vi "BallShear_main.vi"() -> ()   [LabVIEW 2013]
panel:
  out "Livefeed":path
  out "Ball_Detection":path
  out "Coord_Conversion":path
  out "VCoord":path
  out "RCoord":path
  out "Force Reading":path
  out "Analyzed Image":path
  out "Package Image":path
  out "Default Image":path
  in  "Array":dbl[][](array[numeric])
  out "Selected \nCoordinates":dbl[][](array[numeric])
  out "Selected Indices":dbl[](array[numeric])
  out "Coordinates":dbl[][](array[numeric])
  out "Ball IDs":string[](array[string])
  out "Current Step":i32
  in  "Options":enum32{"Shear", "Results", "Settings"}(tab)
  out "Status":string
  out "# Balls Selected":dbl
  in  "Shear Speed":dbl=1.0 min=1.0 max=2.0 step=0.01 format="%#_6f"
  out "Total Steps":dbl
  in  "Check":bool
  out "Ready":bool
  in  "Remove Package":bool
  in  "Proceed":bool
  in  "Preceed":bool
  out "Step":dbl
  out "Package":picture
  in  "Ball Selection":i32[](listbox)
  in  "Max Shear Speed":dbl
  in  "Min Shear Speed":dbl
  in  "Image Path":path
  in  "Image Name":string
  out "Displayed Image":path=path "C:/Users/nsliwa/Documents/GitHub/Ball_Shear/Images/default.jpg"
  in  "Image Path":string
  out "Ready":bool
  in  "Power":bool=TRUE
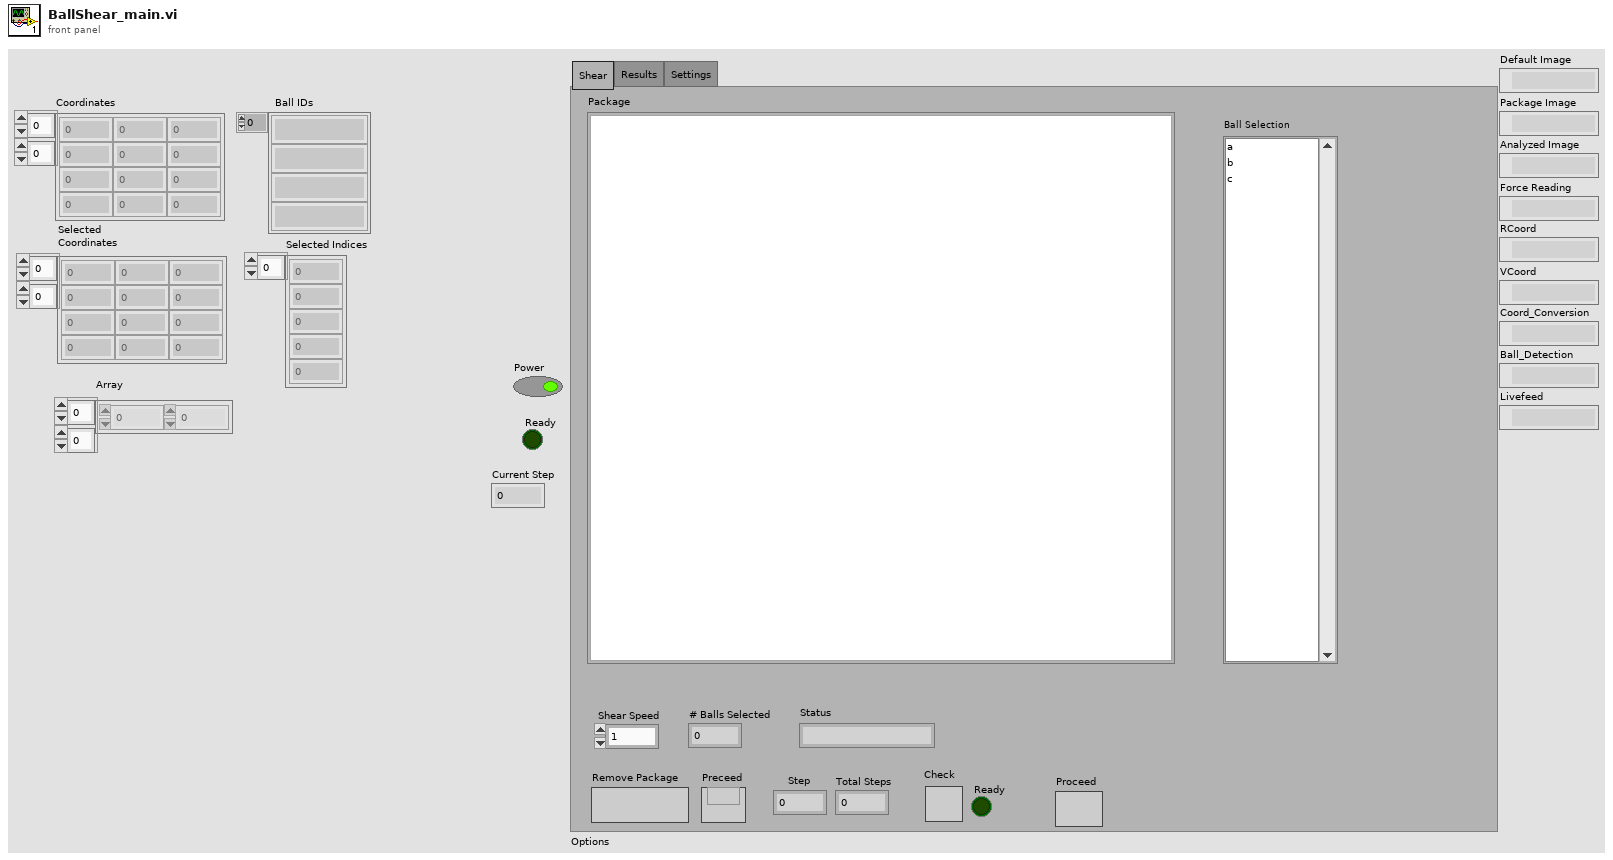
[diagram p1: front panel]
types:
  T1 = typedef "imagedata.ctl" = cluster{"image type":i32, "image depth":i32, "image":u8[], "mask":u8[], "colors":u32[], "Rectangle":cluster{"left":i16, "top":i16, "right":i16, "bottom":i16}}
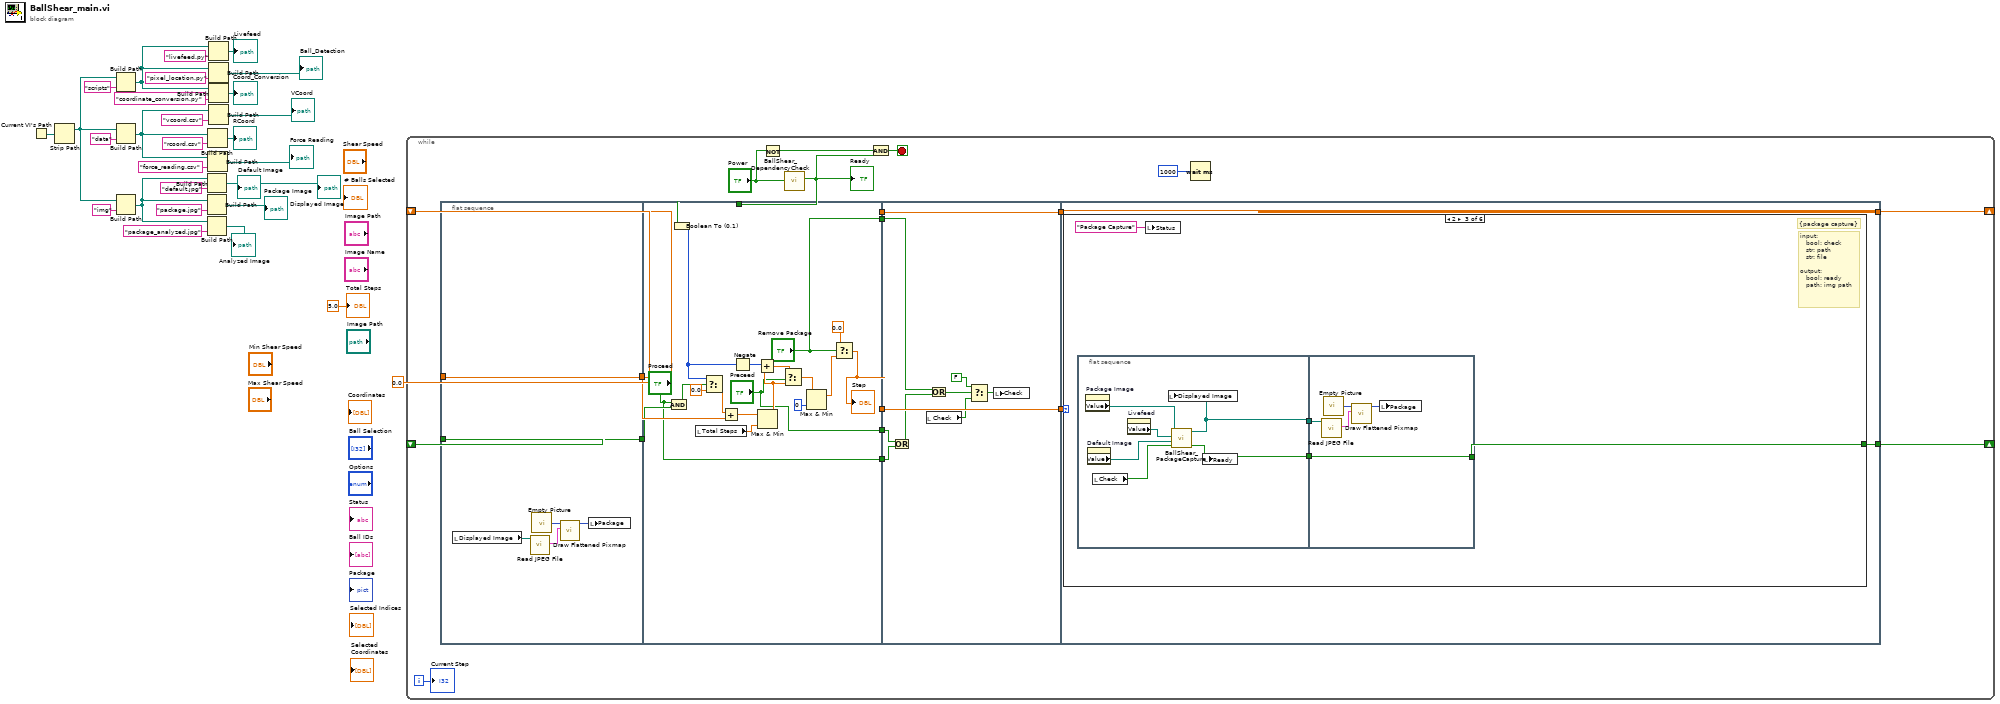
[diagram p0: block diagram]
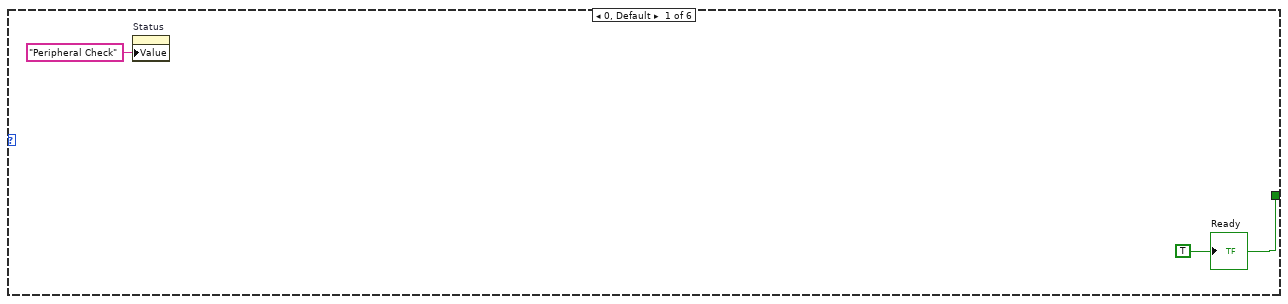
[diagram p2: hidden frame]
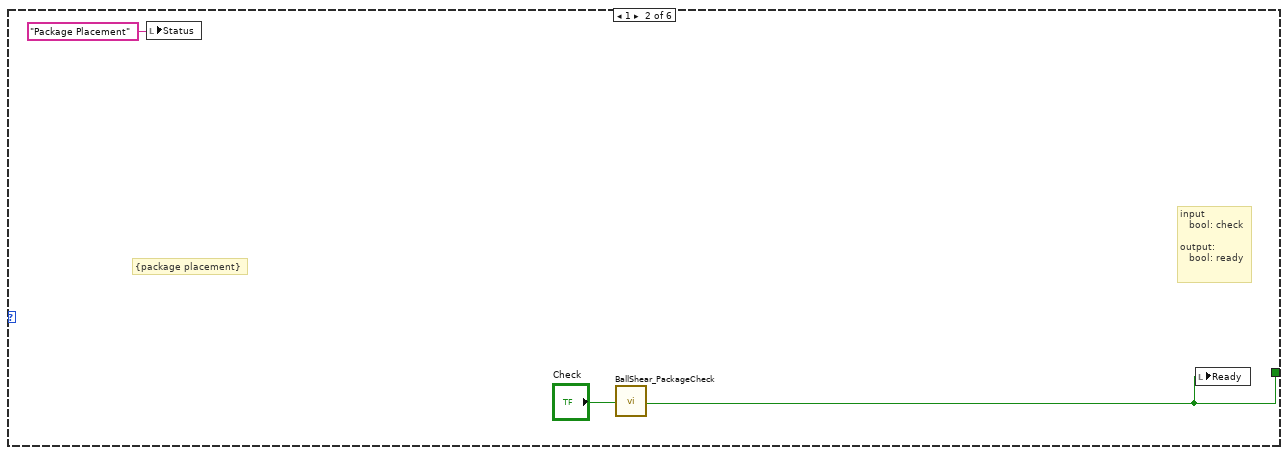
[diagram p3: hidden frame]
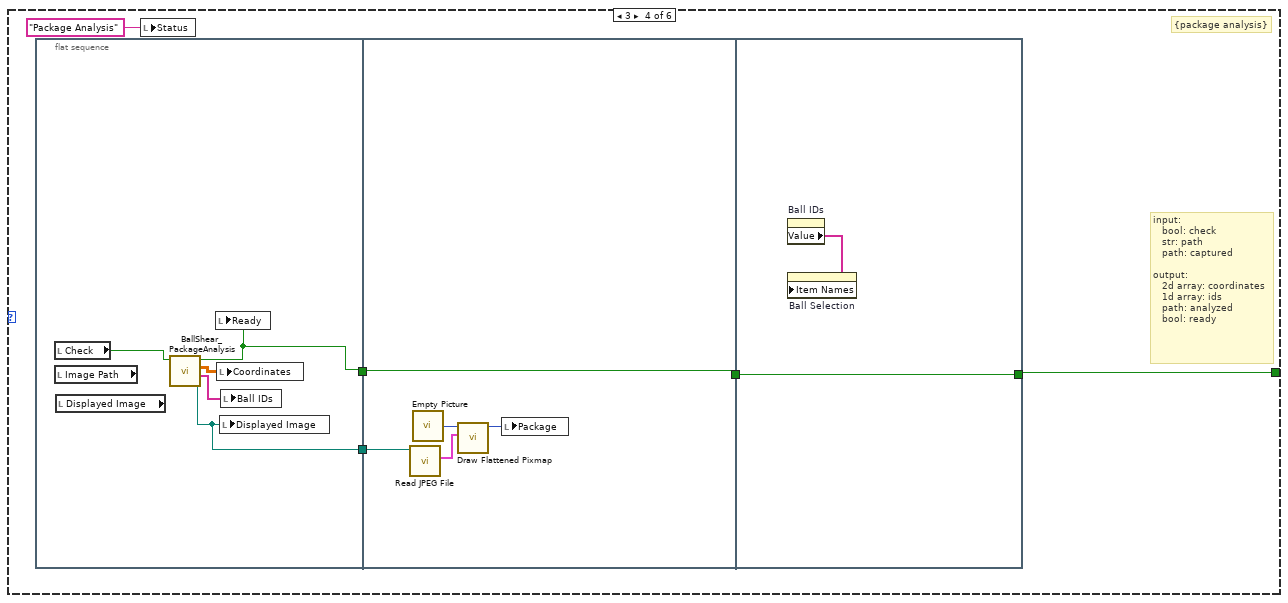
[diagram p4: hidden frame]
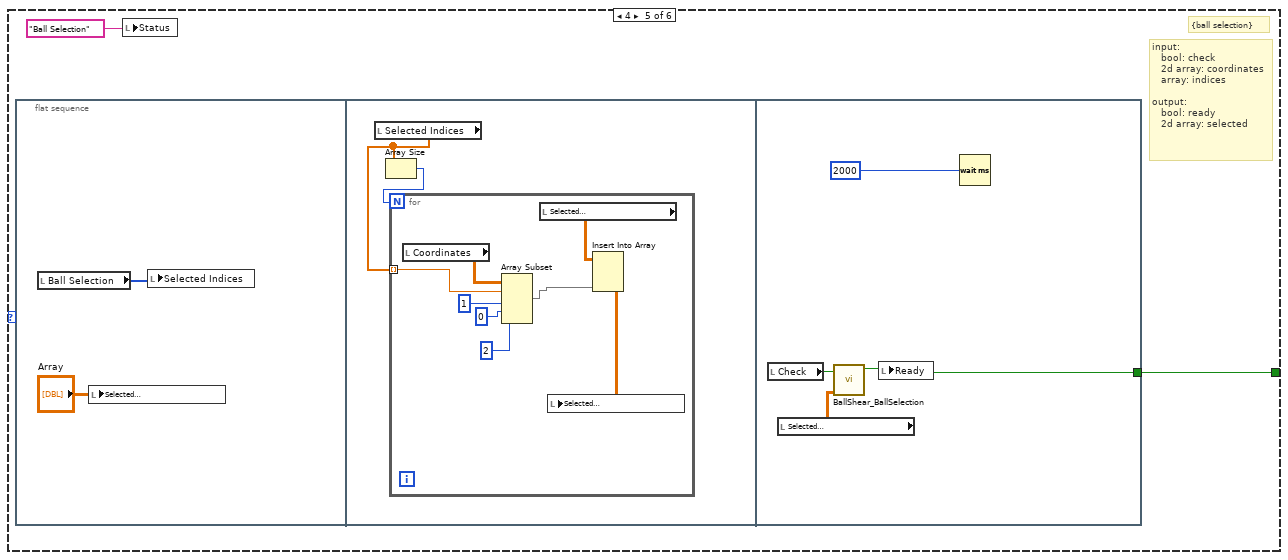
[diagram p5: hidden frame]
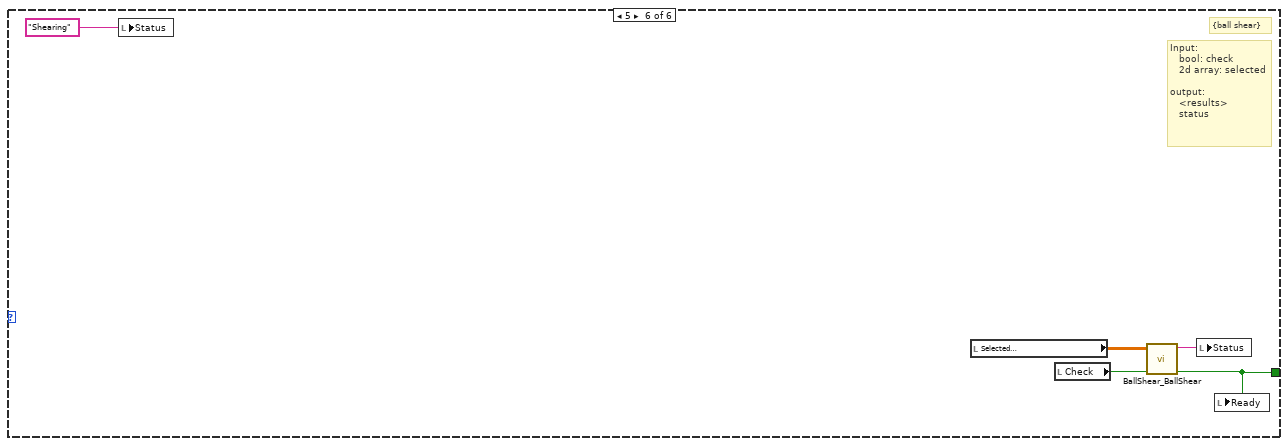
[diagram p6: hidden frame]
diagram:
  n1 = Current VI's Path() -> (path=w26:path)
  n2 = Strip Path(path=w26) -> (stripped path=w24:path)  [unwired: 1 out]
  n3 = Build Path(base path=w24, name or relative path="scripts") -> (appended path=w20:path)
  n4 = Build Path(base path=w24, name or relative path="data") -> (appended path=w15:path)
  n5 = Build Path(base path=w24, name or relative path="img") -> (appended path=w21:path)
  n6 = Build Path(base path=w21, name or relative path="default.jpg") -> (appended path=→"Displayed Image" →"Default Image":path)
  n7 = Build Path(base path=w21, name or relative path="package.jpg") -> (appended path=→"Package Image":path)
  n8 = Build Path(base path=w21, name or relative path="package_analyzed.jpg") -> (appended path=→"Analyzed Image":path)
  n9 = Build Path(base path=w15, name or relative path="rcoord.csv") -> (appended path=→"RCoord":path)
  n10 = Build Path(base path=w15, name or relative path="force_reading.csv") -> (appended path=→"Force Reading":path)
  n11 = Build Path(base path=w20, name or relative path="livefeed.py") -> (appended path=→"Livefeed":path)
  n12 = Build Path(base path=w20, name or relative path="pixel_location.py") -> (appended path=→"Ball_Detection":path)
  n13 = Build Path(base path=w20, name or relative path="coordinate_conversion.py") -> (appended path=→"Coord_Conversion":path)
  n14 = Build Path(base path=w15, name or relative path="vcoord.csv") -> (appended path=→"VCoord":path)
  n15 = while {
    shift-right: [w40] -> _
    shift-left: 0.0 ("Step") -> [w42]
    shift-right: [w38] -> _
    shift-left: _ -> [w36]
    i -> [w43]
    stop <- w45 stop-if-true
    n16 = flat-sequence {
      tunnel: w42 -> [w53]
      tunnel: [w53] -> w39
      tunnel: [w52] -> w37
      tunnel: w36 -> [w52]
      tunnel: w41 -> [w68]
      tunnel: [w59] -> w35
      tunnel: w39 -> [w69]
      tunnel: [w59] -> w33
      tunnel: w37 -> [w58]
      tunnel: ["Remove Package"] -> w31
      tunnel: ["Proceed"] -> w30
      tunnel: ["Preceed"] -> w29
      tunnel: w35 -> [w83]
      tunnel: [w83] -> w34
      tunnel: w33 -> [w82]
      tunnel: [w82] -> w32
      tunnel: w31 -> [w79]
      tunnel: w30 -> [w80]
      tunnel: w29 -> [w81]
      tunnel: [w86] -> w40
      tunnel: w34 -> [w86]
      tunnel: w32 -> [w85]
      tunnel: [w84] -> w38
      frame #0 {
        n17 = local read "Displayed Image"() -> (w48:path)
        n18 = call <vilib>:"Read JPEG File.vi"("path to JPEG file"=w48) -> ("image data"=w49:T1)  [unwired: 8 in, 2 out]
        n19 = call "Empty Picture"() -> ("empty picture"=w50:picture)
        n20 = call <vilib>:"Draw Flattened Pixmap.vi"("image data"=w49, "picture"=w50) -> ("new picture"=w51:picture)  [unwired: 7 in]
        n21 = local write "Package"(w51) -> ()
      }
      frame #1 {
        n22 = And(x="Proceed", y=w58) -> (x .and. y?=w57:bool)
        n23 = Boolean To (0,1)(Boolean=w68) -> (0, 1=w67:i16)
        n24 = local read "Total Steps"() -> (w61:dbl)
        n25 = Select(t=w67, s=w57, f=0.0) -> (s? t:f=w71:dbl)
        n26 = Add(x=w71, y=w69) -> (x+y=w66:dbl)
        n27 = Negate(x=w67) -> (-x=w72:i16)
        n28 = Max & Min(x=w66, y=w61) -> (min(x,y)=w65:dbl)  [unwired: 1 out]
        n29 = Add(x=w72, y=w65) -> (x+y=w73:dbl)
        n30 = Select(t=w73, s="Preceed", f=w65) -> (s? t:f=w64:dbl)
        n31 = Max & Min(x=w64, y=i16 0) -> (max(x,y)=w63:dbl)  [unwired: 1 out]
        n32 = Select(t=0.0, s="Remove Package", f=w63) -> (s? t:f=w59:dbl)
        "Step" <- w59
      }
      frame #2 {
        n33 = Or(x=w81, y=w80) -> (x .or. y?=w78:bool)
        n34 = local read "Check"() -> (w75:bool)
        n35 = Or(x=w79, y=w78) -> (x .or. y?=w77:bool)
        n36 = Select(t=FALSE, s=w77, f=w75) -> (s? t:f=w74:bool)
        n37 = local write "Check"(w74) -> ()
      }
      frame #3 {
        n38 = case shown="2" w85 {
          tunnel: [w88 w90 w94 w110 w124 w144] -> w84
          frame 0, Default {
            w88 = TRUE
            n39 = property on="Status" class="Str"("Value"="Peripheral Check" ("Status")) -> ()  [unwired: 2 in, 2 out]
            "Ready" <- w88
          }
          frame 1 {
            # "input\n   bool: check\n\noutput:\n   bool: ready"
            # "{package placement}"
            n40 = local write "Status"("Package Placement" ("Status")) -> ()
            n41 = call "BallShear_PackageCheck.vi"("Check"="Check") -> ("Ready"=w90:bool)  [unwired: 10 in]
            n42 = local write "Ready"(w90) -> ()
          }
          frame 2 {
            # "input: \n   bool: check\n   str: path\n   str: file\n\noutput:\n   bool: ready\n   path: img path"
            # "{package capture}"
            n43 = flat-sequence {
              tunnel: [w101] -> w93
              tunnel: [w100] -> w92
              tunnel: w93 -> [w106]
              tunnel: w92 -> [w103]
              tunnel: [w106] -> w94
              frame #0 {
                n44 = property on="Package Image" class="Path"() -> ("Value"=w98:path)  [unwired: 2 in, 2 out]
                n45 = property on="Default Image" class="Path"() -> ("Value"=w96:path)  [unwired: 2 in, 2 out]
                n46 = local read "Check"() -> (w99:bool)
                n47 = property on="Livefeed" class="Path"() -> ("Value"=w97:path)  [unwired: 2 in, 2 out]
                n48 = call "BallShear_PackageCapture.vi"("Capture"=w99, "Default Image Path"=w96, "Python Script Path"=w97, "Target Image Path"=w98) -> ("Success"=w101:bool, "Actual Image Path"=w100:path)  [unwired: 6 in]
                n49 = local write "Displayed Image"(w100) -> ()
                n50 = local write "Ready"(w101) -> ()
              }
              frame #1 {
                n51 = call <vilib>:"Read JPEG File.vi"("path to JPEG file"=w103) -> ("image data"=w105:T1)  [unwired: 8 in, 2 out]
                n52 = call "Empty Picture"() -> ("empty picture"=w104:picture)
                n53 = call <vilib>:"Draw Flattened Pixmap.vi"("image data"=w105, "picture"=w104) -> ("new picture"=w102:picture)  [unwired: 7 in]
                n54 = local write "Package"(w102) -> ()
              }
            }
            n55 = local write "Status"("Package Capture" ("Status")) -> ()
          }
          frame 3 {
            # "input:\n   bool: check\n   str: path\n   path: captured\n\noutput:\n   2d array: coordinates\n   1d array: ids\n   path: analyzed\n   bool: ready"
            # "{package analysis}"
            n56 = flat-sequence {
              tunnel: [w113] -> w109
              tunnel: [w112] -> w108
              tunnel: w109 -> [w121]
              tunnel: w108 -> [w117]
              tunnel: [w121] -> w107
              tunnel: [w123] -> w110
              tunnel: w107 -> [w123]
              frame #0 {
                n57 = local read "Check"() -> (w116:bool)
                n58 = local read "Image Path"() -> ()  [unwired: 1 out]
                n59 = local read "Displayed Image"() -> ()  [unwired: 1 out]
                n60 = call "BallShear_PackageAnalysis.vi"("Analyze"=w116) -> ("Displayed Path"=w112:path, "IDs"=w114:string[], "Coordinates"=w115:dbl[][], "Success"=w113:bool)  [unwired: 7 in]
                n61 = local write "Ready"(w113) -> ()
                n62 = local write "Coordinates"(w115) -> ()
                n63 = local write "Displayed Image"(w112) -> ()
                n64 = local write "Ball IDs"(w114) -> ()
              }
              frame #1 {
                n65 = call <vilib>:"Read JPEG File.vi"("path to JPEG file"=w117) -> ("image data"=w120:T1)  [unwired: 8 in, 2 out]
                n66 = call "Empty Picture"() -> ("empty picture"=w119:picture)
                n67 = call <vilib>:"Draw Flattened Pixmap.vi"("image data"=w120, "picture"=w119) -> ("new picture"=w118:picture)  [unwired: 7 in]
                n68 = local write "Package"(w118) -> ()
              }
              frame #2 {
                n69 = property on="Ball IDs" class="Arr (strict)"() -> ("Value"=w122:string[])  [unwired: 2 in, 2 out]
                n70 = property on="Ball Selection" class="LstBox (strict)"("Item Names"=w122) -> ()  [unwired: 2 in, 2 out]
              }
            }
            n71 = local write "Status"("Package Analysis" ("Status")) -> ()
          }
          frame 4 {
            # "input:\n   bool: check\n   2d array: coordinates\n   array: indices\n\noutput: \n   bool: ready\n   2d array: selected"
            # "{ball selection}"
            n72 = flat-sequence {
              tunnel: [w139] -> w124
              frame #0 {
                n73 = local read "Ball Selection"() -> (w127:i32[])
                n74 = local write "Selected \nCoordinates"("Array") -> ()
                n75 = local write "Selected Indices"(w127) -> ()
              }
              frame #1 {
                n76 = local read "Selected Indices"() -> (w128:dbl[])
                n77 = Array Size(array=w128) -> (size(s)=w129:i32)
                n78 = for {
                  N: w129 -> [_]
                  tunnel: w128 -> [w132] mode=indexing
                  n79 = local read "Coordinates"() -> (w136:dbl[][])
                  n80 = Array Subset(array=w136, index (row)=w132, length (row)=1 ("length"), index (col)=0 ("index"), length (col)=2 ("length")) -> (w133:dbl[][])
                  n81 = local read "Selected \nCoordinates"() -> (w137:dbl[][])
                  n82 = Insert Into Array(array=w137, new element=w133) -> (w130:dbl[][])  [unwired: 2 in]
                  n83 = local write "Selected \nCoordinates"(w130) -> ()
                }
              }
              frame #2 {
                n84 = local read "Check"() -> (w140:bool)
                n85 = local read "Selected \nCoordinates"() -> (w138:dbl[][])
                n86 = call "BallShear_BallSelection.vi"("Selected Balls"=w138, "Check"=w140) -> ("Ready"=w139:bool)  [unwired: 9 in]
                n87 = local write "Ready"(w139) -> ()
                n88 = Wait (ms)(milliseconds to wait=u32 2000) -> ()  [unwired: 1 out]
              }
            }
            n89 = local write "Status"("Ball Selection" ("Status")) -> ()
          }
          frame 5 {
            # "Input: \n   bool: check\n   2d array: selected\n\noutput: \n   <results>\n   status"
            # "{ball shear}"
            n90 = local write "Status"("Shearing" ("Status")) -> ()
            n91 = local read "Selected \nCoordinates"() -> (w143:dbl[][])
            n92 = local read "Check"() -> (w145:bool)
            n93 = call "BallShear_BallShear.vi"("Check"=w145, "Selected Balls"=w143) -> ("Ready"=w144:bool, "Status"=w142:string)  [unwired: 8 in]
            n94 = local write "Status"(w142) -> ()
            n95 = local write "Ready"(w144) -> ()
          }
        }
      }
    }
    n96 = Not(x="Power") -> (.not. x?=w46:bool)
    n97 = call "BallShear_DependencyCheck.vi"("Power"="Power") -> ("Ready"=w41:bool)  [unwired: 10 in]
    "Ready" <- w41
    n98 = And(x=w46, y=w41) -> (x .and. y?=w45:bool)
    n99 = Wait (ms)(milliseconds to wait=u32 1000) -> ()  [unwired: 1 out]
    "Current Step" <- w43
  }
  "Total Steps" <- 5.0 ("Total Steps")
